vi "GE 5565PIORC.DMA.Get Transfer Components.vi"   [LabVIEW 2016, in "GE 5565PIORC.lvclass"]
doc: "Returns the components of a <b>DMA Transfer Spec</b> cluster."
uses:
  GE 5565PIORC.lvclass
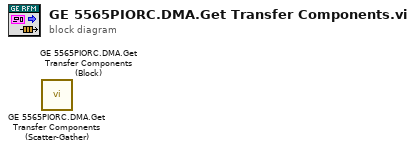
[diagram p0: block diagram]
diagram:
  n1 = call "GE 5565PIORC.DMA.Get Transfer Components (Scatter-Gather).vi"() -> ()  [unwired: 8 in, 4 out]
  n2 = call "GE 5565PIORC.DMA.Get Transfer Components (Block).vi"() -> ()  [unwired: 8 in, 4 out]
